vi "Channel String to details.vi"(11 "String":string) -> (2 "Channel":i32, 3 "Module":i32)   [LabVIEW 2019, in "DAQ970.lvlib" / "DAQ970.lvclass"]
uses:
  Library/DAQ970.lvclass
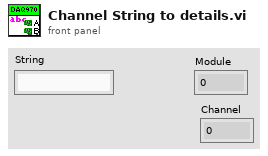
[diagram p1: front panel]
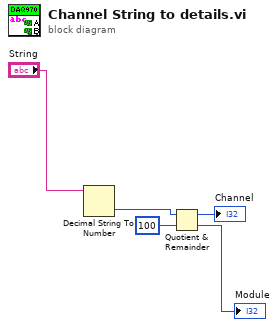
[diagram p0: block diagram]
diagram:
  n1 = Decimal String To Number(string="String") -> (number=w4:i32)  [unwired: 2 in, 1 out]
  n2 = Quotient & Remainder(x=w4, y=100) -> (x-y*floor(x/y)=→"Channel":i32, floor(x/y)=→"Module":i32)
